vi "Prepare Elves.vi"(1 "Elves' Sonar":bool[][](array[boolean])) -> (0 "Elves":set{T1}(c389))   [LabVIEW 2020, in "AoC 2022.lvlib"]
uses:
  AoC 2022.lvlib
  Day 15 - Beacon Exclusion Zone/private/Location.ctl
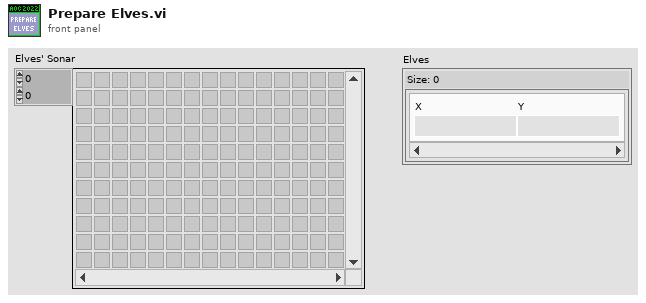
[diagram p1: front panel]
types:
  T1 = typedef "AoC 2022.lvlib/Location.ctl" = cluster{"X":i32, "Y":i32}
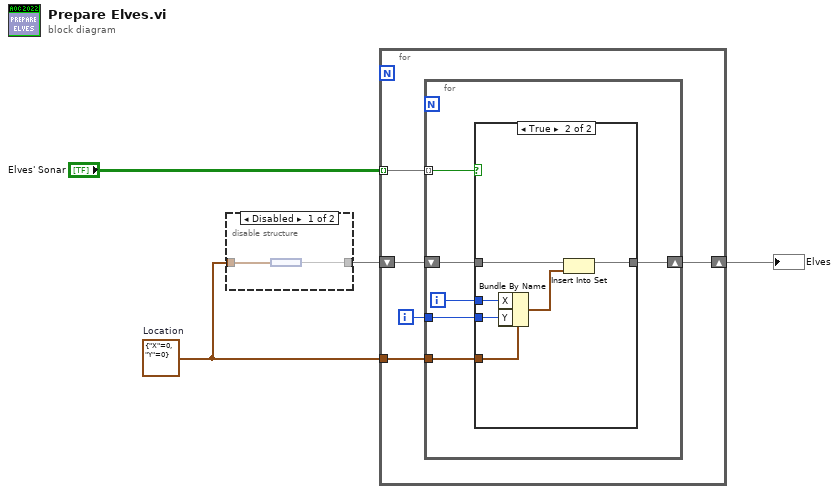
[diagram p0: block diagram]
diagram:
  w1 = T1 {"X"=0, "Y"=0}  # Location
  n1 = disable-structure shown="Disabled" {
    disable-tunnel: [w6 _] -> w2
    disable-tunnel: w1 -> [w5 _]
    frame Disabled {
      n2 = node(w5) -> (w6:set{T1})
    }
    frame Enabled {
    }
  }
  n3 = for {
    tunnel: "Elves' Sonar" -> [w9] mode=indexing
    shift-right: [w11] -> w3
    shift-left: w2 -> [w10]
    tunnel: w1 -> [w8]
    i -> [w7]
    n4 = for {
      shift-right: [w16] -> w11
      shift-left: w10 -> [w17]
      tunnel: w9 -> [w12] mode=indexing
      tunnel: w8 -> [w15]
      tunnel: w7 -> [w13]
      i -> [w14]
      n5 = case shown="True" w12 {
        tunnel: w17 -> [w18 w21]
        tunnel: [w18 w20] -> w16
        tunnel: w15 -> [_ w24]
        tunnel: w14 -> [_ w23]
        tunnel: w13 -> [_ w22]
        frame False {
        }
        frame True {
          n6 = Bundle By Name(cluster=w24, "X"=w23, "Y"=w22) -> (w19:T1)
          n7 = Insert Into Set(10:w19, 11:w21) -> (3:w20:set{T1})  [unwired: 1 out]
        }
      }
    }
  }
  "Elves" <- w3
